vi "AlliGator Unzip Python Plugins.vi"(8 "Error In":errorcluster, 11 "Application Directory":path) -> (0 "Error Out":errorcluster, 3 "Python Plugins Folder":path)   [LabVIEW 2021, in "AlliGator Python Plugins.lvlib"]
doc: "Unzips python plugin archive provided with AlliGator installation."
uses:
  AlliGator Python Plugins.lvlib
  Settings/AlliGator Settings List.ctl
  Globals, Variables, Constants/AlliGator Globals.vi
  <userlib>/_OpenG.lib/lvzip/lvzip.llb/subVI/ZLIB Extract File (Path)__ogtk.vi
  <userlib>/_OpenG.lib/lvzip/lvzip.llb/subVI/ZLIB Open Unzip Archive (Path)__ogtk.vi
  Variant/Variant to Data/Variant to String.vi
  Settings/AlliGator Settings.lvlib
  Variant/Variant to Data/Variant to Data.lvlib
  Globals, Variables, Constants/AlliGator Globals, Variables & Constants.lvlib
panel:
  out "Unmodified Files":path[](array[path])
  out "New Files":path[](array[path])
  # "see the AlliGator License on the block diagram (Ctrl+E or Window:Show Block Diagram)"
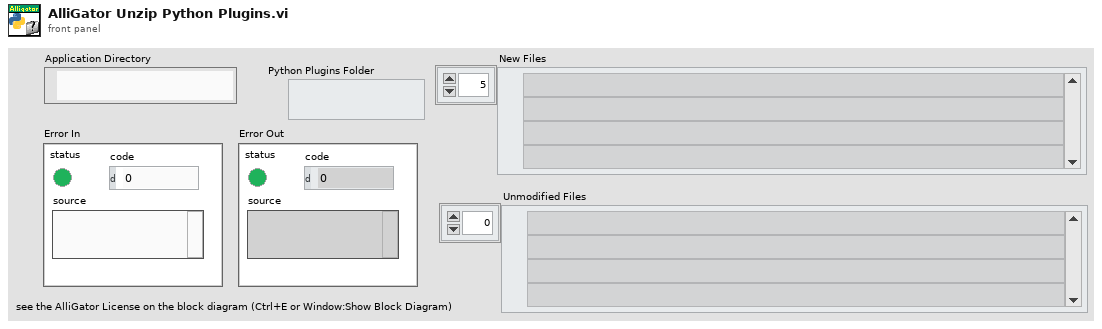
[diagram p1: front panel]
types:
  T1 = typedef "AlliGator Settings.lvlib/AlliGator Settings List.ctl" = enum16{"GUI:Visible Settings Tab", "GUI:Last Run Version", "Source Image:Use Image Histogram for Contrast", "Source Image:Low Count Pixels Rejection Options", "Source Image:High Count Pixels Rejection Options", "Source Image:Use Image Brightness", "Source Image:Blend Overlay with Image Background", "Source Image:Use Fixed ROI Diameter", "Source Image:ROI Diameter", "Source Image:ROI Center Color", "Source Image:Peak Threshold", "Source Image:Intensity Threshold", "Source Image:Image Binning Options", "Source Image:Image Smoothing Options", "Source Image:Image Histogram Active", "Source Image:Invert Binary Mask", "Source Image:Hot Pixel Removal", "Source Image:Overlay Analyzed ROI Center", "Source Image:Auto-Adjust Contrast", "Source Image:Histogram Lower Percentile", "Source Image:Histogram Upper Percentile", "Source Image:Save Source Image", "Source Image:Scale Bar Options", "Source Image:Image Resolution (Pixel Size)", "Source Image:Flatfield Correction", "Source Image:Show Dead Left Columns Correction", "Source Image:Dead Left Columns Correction", "Source Image:Image Pre-Processing Operations Order", "Source Image:Overlay ROI Median", "Source Image:Median Overlay Color", "Data Information:Gate Width", "Data Information:Nanotime Gate Separation", "Data Information:Macrotime Gate Separation", "Data Information:Gate Step", "Data Information:# Gates", "Data Information:Gate Image Exposure", "Data Information:Gate Image Integration", "Data Information:Gates to Skip", "Data Information:Gates to Keep", "Data Information:Define Gates to", "Data Information:Channel Name", "Data Information:Available Channel Names", "Data Information:Channel Arithmetic", "Data Information:Background File Subtraction", "Data Information:Background File", "Data Information:Background Scaling Factor", "Data Information:Background Pile-up Correction", "Data Information:Background Pixel Well Capacity", "Data Information:Laser Period", "Data Information:SYNC Period", "Data Information:Pile-up Correction", "Data Information:Pixel Well Capacity", "Data Information:Dataset Scaling Factor", "Fluorescence Decay_Decay Pre-Processing:Reverse Gates", "Fluorescence Decay_Decay Pre-Processing:Verbose Decay Pre-Processing", "Fluorescence Decay_Decay Pre-Processing:Use Decay Pre-Processing", "Fluorescence Decay_Decay Pre-Processing:Background Subtraction", "Fluorescence Decay_Decay Pre-Processing:Background Definition Range", "Fluorescence Decay_Decay Pre-Processing:Baseline Subtraction Method", "Fluorescence Decay_Decay Pre-Processing:Decay Pre-Processing Operations Order", "Fluorescence Decay_Decay Pre-Processing:Smoothing Parameter", "Fluorescence Decay_Decay Pre-Processing:Shift Decay", "Fluorescence Decay_Decay Pre-Processing:Decay Shift Parameters", "Fluorescence Decay_Decay Pre-Processing:Fold Decay", "Fluorescence Decay_Decay Pre-Processing:# Folds", "Fluorescence Decay_Decay Pre-Processing:1-Normalize Decay", "Fluorescence Decay_Decay Pre-Processing:[0-1]-Normalize Decay", "Fluorescence Decay_Decay Pre-Processing:Smoothen Decay", "Fluorescence Decay_Decay Pre-Processing:Extrapolate Decay", "Fluorescence Decay_Decay Pre-Processing:Use Periodicity", "Fluorescence Decay_Decay Pre-Processing:Use Cursors", "Fluorescence Decay_Decay Pre-Processing:Tail Fraction", "Fluorescence Decay_Decay Pre-Processing:Head Fraction", "Fluorescence Decay_Decay Pre-Processing:Additional Points", "Fluorescence Decay_Decay Pre-Processing:Straighten Decay", "Fluorescence Decay_Decay Pre-Processing:Constant Background", "Fluorescence Decay_Decay Pre-Processing:Pixel-Normalize Decay", "Fluorescence Decay_Advanced Analysis:Extract IRF instead of Decay", "Fluorescence Decay_Advanced Analysis:IRF Extraction Options", "Fluorescence Decay_Advanced Analysis:IRF Optimization Options", "Fluorescence Decay_Advanced Analysis:Square Pulse Options", "Fluorescence Decay_Advanced Analysis:IRF Order", "Fluorescence Decay_Advanced Analysis:IRF Time Constants", "Fluorescence Decay_Advanced Analysis:Wavelet Analysis Options", "Fluorescence Decay_Advanced Analysis:Average Lifetime Options", "Fluorescence Decay_Fit Options:Fit Options", "Fluorescence Decay_Fit Options:Use Legacy Fitting Approach", "Fluorescence Decay_Fit Options:Use Data Information Laser Period", "Fluorescence Decay_Fit Parameters:Displayed Fit Parameters", "Fluorescence Decay_Fit Parameters:Fit Parameter Constraints", "Fluorescence Decay_Fit Parameters:Export Tabulated Results", "Fluorescence Decay_Fit Parameters:MLE Baseline Offset Type", "Fluorescence Decay_Fit Parameters:MLE Baseline Offset", "Fluorescence Decay_Fit Parameters:Guess Parameter Names", "Fluorescence Decay_Fit Parameters:Guess Parameter Values", "Fluorescence Decay_Fit Parameters:Guess Parameters Options", "Fluorescence Decay_Styles:Show Last Decay Only", "Fluorescence Decay_Styles:Decay Graph Color Array", "Fluorescence Decay:Decay Graph Active", "Fluorescence Decay Statistics:Min Peak Value", "Fluorescence Decay Statistics:Reject Low Decay Peak Pixels", "Fluorescence Decay Statistics:Reject High Decay Peak Pixels", "Fluorescence Decay Statistics:Max Peak Value", "Time Traces:Use File Timestamp", "Time Traces:Time Step", "Time Traces:Use Intensity Correction File", "Time Traces:Intensity Correction File", "Phasor Plot:Phasor Plot Smoothing Options", "Phasor Plot:Phasor Plot Size", "Phasor Plot:Phasor Plot Graphics Options", "Phasor Plot:Cumulative Phasor Plot", "Phasor Plot:Use Phasor Brightness", "Phasor Plot:Blend Overlay with Phasor Background", "Phasor Plot:Save Phasor Plot", "Phasor Plot:Show References", "Phasor Plot:Phasor Ratio Decay Range", "Phasor Plot:Exponential Fading", "Phasor Plot:Phasor Ratio Reference Colors", "Phasor Plot:Reference Radius", "Phasor Plot:Show Color Map Vertices", "Phasor Plot:Phasor Plot Active", "Phasor Plot:Phasor Ratio Color Map Type", "Phasor Plot:Phasor Ratio Color Map", "Phasor Plot:Phasor Ratio Display Range", "Phasor Plot:Selected Image ROI(s)", "Phasor Plot:All Image ROIs", "Phasor Plot:Selected Phasor Plot ROI(s)", "Phasor Plot:All Phasor Plot ROIs", "Phasor Plot:Phasor Ratio Color-Coded Quantity", "Phasor Plot:Store Phasor Harmonics", "Phasor Plot:Draw Reference Segment", "Phasor Plot:User-Defined Quantity", "Phasor Graph:Phasor Frequency", "Phasor Graph:Phasor Ratio Type", "Phasor Graph:Pixel-level Phasor Computation", "Phasor Graph:Save Phasor Graph", "Phasor Graph:Phasor Graph Active", "Phasor Graph:Phasor SDV Options", "Phasor Calibration:Use Backup Calibration if needed", "Phasor Graph:Define Shortest Lifetime as", "Phasor Calibration:Backup Calibration Type", "Phasor Calibration:Calibration Type", "Phasor Calibration:Calibration Lifetime", "Phasor Calibration:Calibration Map Algorithm", "Single-Exponential Phasor Locus (SEPL):Gate Parameters", "Single-Exponential Phasor Locus (SEPL):User-defined Gate", "Single-Exponential Phasor Locus (SEPL):User-defined IRF", "Single-Exponential Phasor Locus (SEPL):Phasor Parameters", "Single-Exponential Phasor Locus (SEPL):Decay & IRF Parameters", "Single-Exponential Phasor Locus (SEPL):Display Parameters", "Lifetime Analysis:Decay Analysis Parameters", "Lifetime Analysis:Lifetime Map Active", "Plugins:Python Settings", "Miscellaneous:Verbose Mode", "Miscellaneous:Beep after Script", "Miscellaneous:Saved Image File Format", "Miscellaneous:Exported Gate Image Settings", "Miscellaneous:Include Loading in Timing", "Miscellaneous:Verbose Settings Mode", "Miscellaneous:Histogram Options", "Miscellaneous:Beep on Error", "Miscellaneous:# Logical Processors Used", "Miscellaneous:ROI Description Max Characters", "Miscellaneous:Verbose Error Mode", "Miscellaneous:Transparent Mask Color"}
  T2 = typedef "ZLIB Unzip Handle__ogtk.ctl" = refnum<k1>
  T3 = typedef "ZLIB File Info__ogtk.ctl" = cluster{"version":u32, "version needed":u32, "encrypted":bool, "flag":u32, "compression":i32, "dos date":u32, "crc":u32, "compressed size":i64, "uncompressed size":i64, "file comment":string, "disk num start":u32, "internal fa":u32, "external fa":u32, "file timestamp":u32, "extra info records":cluster{"id":u16, "data":u8[]}[]}
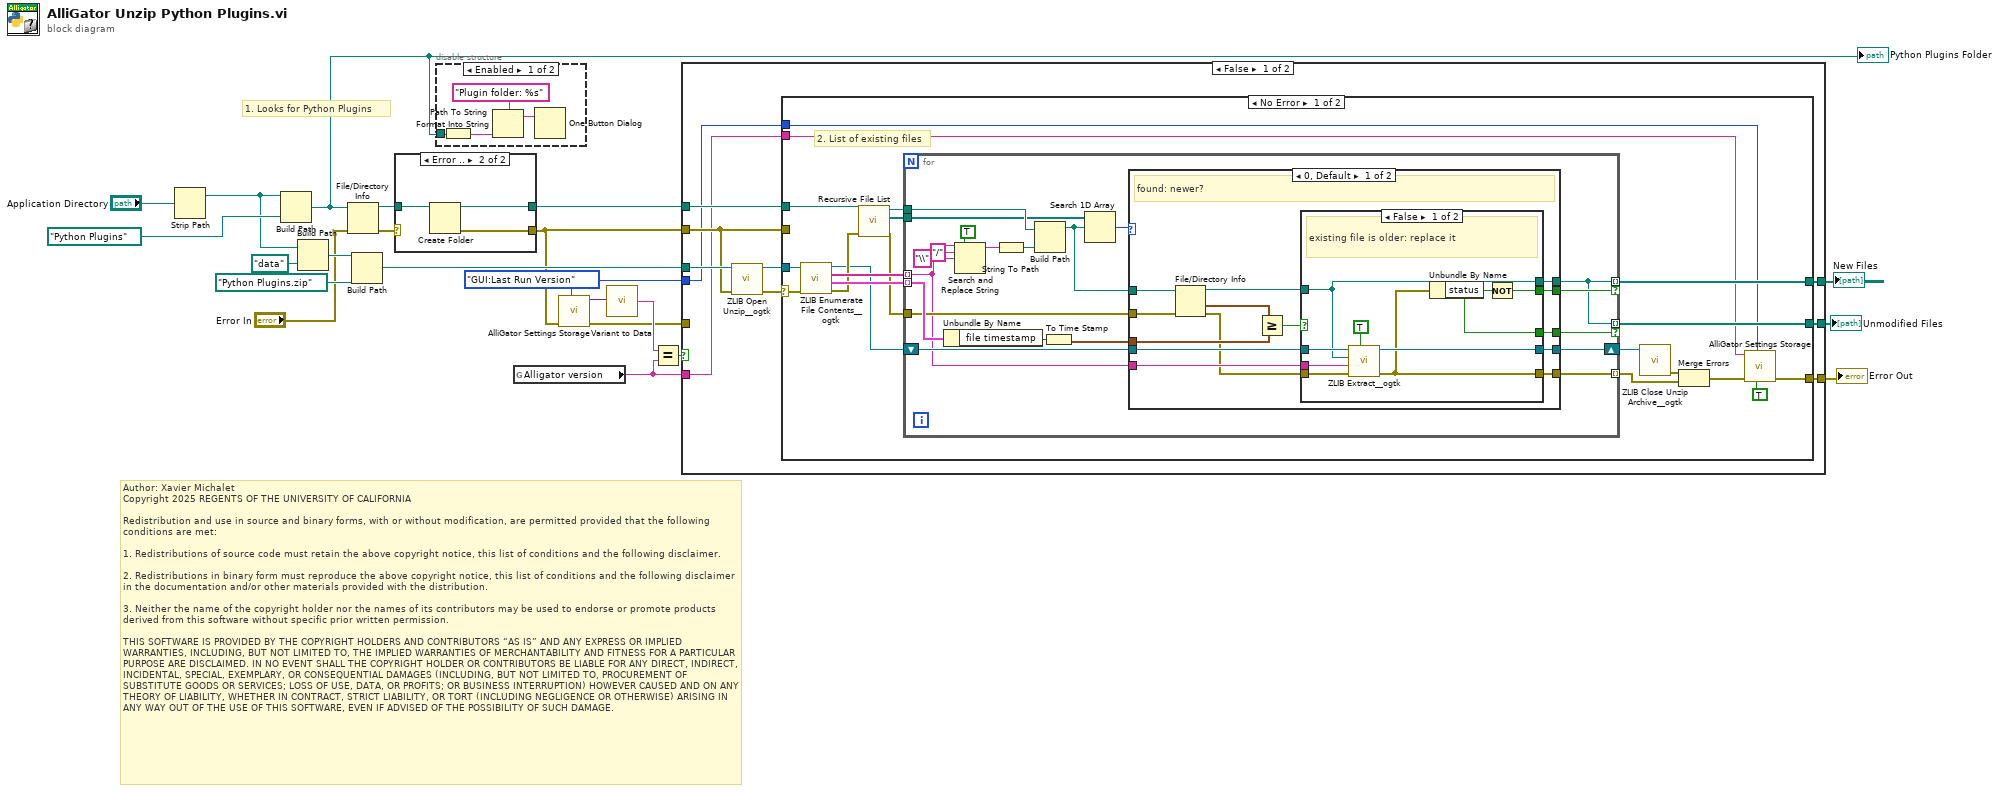
[diagram p0: block diagram]
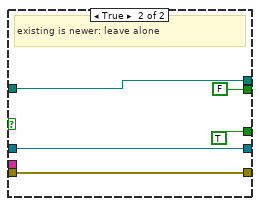
[diagram p3: hidden frame]
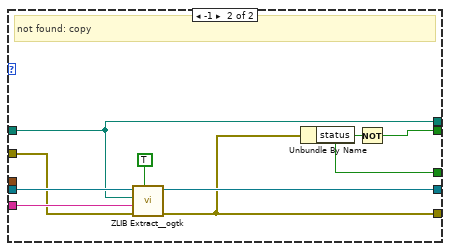
[diagram p4: hidden frame]
diagram:
  w4 = AlliGator_Settings_List."GUI:Last Run Version" ("AlliGator Settings List")
  # "Author: Xavier Michalet\nCopyright 2025 REGENTS OF THE UNIVERSITY OF CALIFORNIA\n\nRedistribution and use in source and binary forms, with or without modification, are permitted provided that the following conditions are met:\n\n1. Redistributions of source code must retain the above copyright notice, this list of conditions and the following disclaimer.\n\n2. Redistributions in binary form must reproduce the above copyright notice, this list of conditions and the following disclaimer in the documentation and/or other materials provided with the distribution.\n\n3. Neither the name of the copyright holder nor the names of its contributors may be used to endorse or promote products derived from this software without specific prior written permission.\n\nTHIS SOFTWARE IS PROVIDED BY THE COPYRIGHT HOLDERS AND CONTRIBUTORS “AS IS” AND ANY EXPRESS OR IMPLIED WARRANTIES, INCLUDING, BUT NOT LIMITED TO, THE IMPLIED WARRANTIES OF MERCHANTABILITY AND FITNESS FOR A PARTICULAR PURPOSE ARE DISCLAIMED. IN NO EVENT SHALL THE COPYRIGHT HOLDER OR CONTRIBUTORS BE LIABLE FOR ANY DIRECT, INDIRECT, INCIDENTAL, SPECIAL, EXEMPLARY, OR CONSEQUENTIAL DAMAGES (INCLUDING, BUT NOT LIMITED TO, PROCUREMENT OF SUBSTITUTE GOODS OR SERVICES; LOSS OF USE, DATA, OR PROFITS; OR BUSINESS INTERRUPTION) HOWEVER CAUSED AND ON ANY THEORY OF LIABILITY, WHETHER IN CONTRACT, STRICT LIABILITY, OR TORT (INCLUDING NEGLIGENCE OR OTHERWISE) ARISING IN ANY WAY OUT OF THE USE OF THIS SOFTWARE, EVEN IF ADVISED OF THE POSSIBILITY OF SUCH DAMAGE."
  # "1. Looks for Python Plugins"
  n1 = Strip Path(path="Application Directory") -> (stripped path=w2:path)  [unwired: 1 out]
  n2 = Build Path(base path=w2, name or relative path=path "Python Plugins") -> (appended path=w1:path)
  "Python Plugins Folder" <- w1
  n3 = Build Path(base path=w2, name or relative path=path "data") -> (appended path=w21:path)
  n4 = File/Directory Info(path=w1, error in="Error In") -> (path out=w17:path, error out=w18:errorcluster)  [unwired: 5 out]
  n5 = Build Path(base path=w21, name or relative path=path "Python Plugins.zip") -> (appended path=w14:path)
  n6 = case shown="Error .." w18 {
    selector: w18 -> [w23 _]
    tunnel: w17 -> [w24 w27]
    tunnel: [w24 w25] -> w13
    tunnel: [w23 w26] -> w9
    frame No Error {
    }
    frame Error {
      n7 = Create Folder(path (use dialog)=w27) -> (created path=w25:path, error out=w26:errorcluster)  [unwired: 2 in, 1 out]
    }
  }
  n8 = disable-structure shown="Enabled" {
    disable-tunnel: w1 -> [w31 _]
    frame Enabled {
      n9 = Path To String(path=w31) -> (string=w29:string)
      n10 = Format Into String(format string="Plugin folder: %s", w29) -> (resulting string=w30:string)  [unwired: 2 in, 1 out]
      n11 = One Button Dialog(message=w30) -> ()  [unwired: 1 in, 1 out]
    }
    frame Disabled {
    }
  }
  n12 = global read "AlliGator Globals.vi" "Alligator version"() -> (w3:string)
  n13 = call "AlliGator Settings Storage.vi"("AlliGator Settings List"=w4, "Error In"=w9) -> ("Error Out"=w5:errorcluster, "Variant Data out"=w8:variant)  [unwired: 8 in]
  n14 = call-poly "Variant to Data.vi"("Variant"=w8) -> ("String"=w7:string)  [unwired: 8 in]
  n15 = Equal?(x=w7, y=w3) -> (x = y?=w6:bool)
  n16 = case shown="False" w6 {
    tunnel: w14 -> [w39 _]
    tunnel: w13 -> [w38 _]
    tunnel: [w37 _] -> w12
    tunnel: [w36 _] -> w11
    tunnel: [w35 w120] -> w10
    tunnel: w9 -> [w34 _]
    tunnel: w5 -> [_ w120]
    tunnel: w4 -> [w33 _]
    tunnel: w3 -> [w32 _]
    frame False {
      n17 = call-poly <userlib>:"ZLIB Open Unzip__ogtk.vi"("error in (no error)"=w34, "archive name"=w39) -> ("error out"=w41:errorcluster, "unzip Refnum"=w40:T2)  [unwired: 4 in]
      n18 = case shown="No Error" w41 {
        selector: w41 -> [w59 _]
        tunnel: w40 -> [w58 _]
        tunnel: w38 -> [w56 _]
        tunnel: [w51 _] -> w37
        tunnel: [w49 _] -> w36
        tunnel: [w45 w119] -> w35
        tunnel: w34 -> [_ w119]
        tunnel: w33 -> [w44 _]
        tunnel: w32 -> [w43 _]
        frame No Error {
          # "2. List of existing files"
          n19 = call <userlib>:"ZLIB Enumerate File Contents__ogtk.vi"("error in (no error)"=w59, "unzip Refnum"=w58) -> ("error out"=w57:errorcluster, "file infos"=w61:T3[], "file names"=w60:string[], "unzip Refnum out"=w52:T2)  [unwired: 5 in, 1 out]
          n20 = call <vilib>:"Recursive File List.vi"("error in (no error)"=w57, "Folder Path"=w56) -> ("error out"=w53:errorcluster, "All Files in Dir"=w54:path[], "dup Folder Path"=w55:path)  [unwired: 5 in, 2 out]
          n21 = for {
            tunnel: w61 -> [w81] mode=indexing
            tunnel: w60 -> [w67] mode=indexing
            tunnel: w55 -> [w74]
            tunnel: w54 -> [w73]
            tunnel: w53 -> [w70]
            shift-right: [w66] -> w50
            shift-left: w52 -> [w68]
            tunnel: [w65] -> w47 mode=indexing
            tunnel: [w63] -> w51 mode=indexing if=w64
            tunnel: [w63] -> w49 mode=indexing if=w62
            n22 = Unbundle By Name(w81) -> ("file timestamp"=w80:u32)
            n23 = Search and Replace String(replace all?=TRUE ("replace all? (F)"), input string=w67, search string="/", replace string="\\" ("replace string (\"\")")) -> (result string=w79:string)  [unwired: 4 in, 3 out]
            n24 = String To Path(string=w79) -> (path=w75:path)
            n25 = Build Path(base path=w74, name or relative path=w75) -> (appended path=w71:path)
            n26 = To Time Stamp(1:w80) -> (0:w69:timestamp)
            n27 = Search 1D Array(1D array=w73, element=w71) -> (index of element=w72:i32)  [unwired: 1 in]
            n28 = case shown="0, Default" w72 {
              tunnel: w71 -> [w95 w111]
              tunnel: w70 -> [w94 w113]
              tunnel: [w90 w111] -> w63
              tunnel: [w89 w118] -> w64
              tunnel: [w88 w110] -> w62
              tunnel: w69 -> [w87 _]
              tunnel: w68 -> [w86 w117]
              tunnel: w67 -> [w85 w114]
              tunnel: [w83 w116] -> w66
              tunnel: [w82 w112] -> w65
              frame 0, Default {
                # "found: newer?"
                n29 = File/Directory Info(path=w95, error in=w94) -> (path out=w91:path, last mod=w93:timestamp, error out=w84:errorcluster)  [unwired: 4 out]
                n30 = Greater Or Equal?(x=w93, y=w87) -> (x >= y?=w92:bool)
                n31 = case shown="False" w92 {
                  tunnel: w91 -> [w99 w108]
                  tunnel: [w99 w108] -> w90
                  tunnel: [w97 FALSE] -> w89
                  tunnel: [w96 TRUE] -> w88
                  tunnel: w86 -> [w104 w105]
                  tunnel: w85 -> [w103 _]
                  tunnel: w84 -> [w102 w106]
                  tunnel: [w101 w105] -> w83
                  tunnel: [w98 w106] -> w82
                  frame False {
                    # "existing file is older: replace it"
                    n32 = call-poly <userlib>:"ZLIB Extract__ogtk.vi"("overwrite (F)"=TRUE, "error in (no error)"=w102, "internal name (same as target)"=w103, "target path"=w99, "unzip Refnum"=w104) -> ("error out"=w98:errorcluster, "unzip Refnum out"=w101:T2)  [unwired: 2 in, 1 out]
                    n33 = Unbundle By Name(w98) -> ("status"=w96:bool)
                    n34 = Not(x=w96) -> (.not. x?=w97:bool)
                  }
                  frame True {
                    # "existing is newer: leave alone"
                  }
                }
              }
              frame -1 {
                # "not found: copy"
                n35 = call-poly <userlib>:"ZLIB Extract__ogtk.vi"("overwrite (F)"=TRUE, "error in (no error)"=w113, "internal name (same as target)"=w114, "target path"=w111, "unzip Refnum"=w117) -> ("error out"=w112:errorcluster, "unzip Refnum out"=w116:T2)  [unwired: 2 in, 1 out]
                n36 = Unbundle By Name(w112) -> ("status"=w110:bool)
                n37 = Not(x=w110) -> (.not. x?=w118:bool)
              }
            }
          }
          n38 = call <userlib>:"ZLIB Close Unzip Archive__ogtk.vi"("unzip Refnum"=w50) -> ("error out"=w48:errorcluster)  [unwired: 5 in, 1 out]
          n39 = Merge Errors(w48, w47) -> (w46:errorcluster)
          n40 = call "AlliGator Settings Storage.vi"("Get(F)/Set"=TRUE, "AlliGator Settings List"=w44, "Error In"=w46, "Variant Data in"=w43) -> ("Error Out"=w45:errorcluster)  [unwired: 6 in, 1 out]
        }
        frame Error {
        }
      }
    }
    frame True {
      # "Not the first run: do not overwrite Plugins folder"
    }
  }
  "Error Out" <- w10
  "New Files" <- w12
  "Unmodified Files" <- w11
